vi "Save_Scan_macro.vi"(7 "Application":refnum<k7>, 8 "error in (no error)":errorcluster, 9 "InkScape":string, 10 "BMP INK Path":string, 11 "BMP Path":string) -> (0 "error out":errorcluster, 3 "BMP":picture)   [LabVIEW 2016]
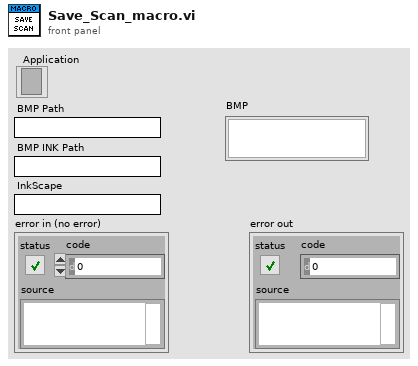
[diagram p1: front panel]
types:
  T1 = cluster{"CenterPosX":dbl, "CenterPosY":dbl, "ImageHeight":dbl, "ImageWidth":dbl}
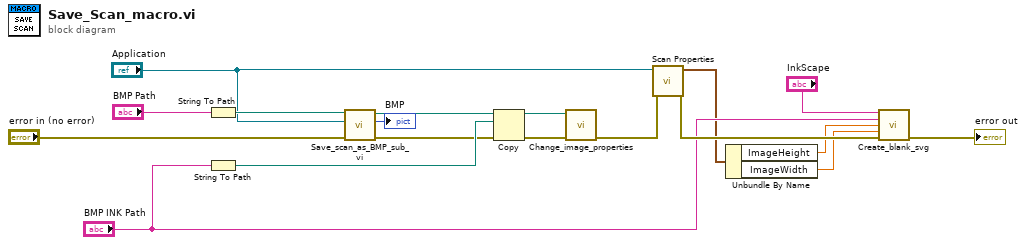
[diagram p0: block diagram]
diagram:
  n1 = String To Path(string="BMP Path") -> (path=w16:path)
  n2 = String To Path(string="BMP INK Path") -> (path=w14:path)
  n3 = call "Save_scan_as_BMP_sub_vi.vi"("error in (no error)"="error in (no error)", "Application"="Application", "BMP Path In"=w16) -> ("Error Out"=w13:errorcluster, "BMP"=→"BMP":picture, "BMP Path Out"=w18:path)  [unwired: 6 in]
  n4 = Copy(8:w13, 10:w14, 11:w18) -> (0:w12:errorcluster, 3:w15:path)  [unwired: 2 in, 1 out]
  n5 = call "Change_image_properties.vi"("error in (no error)"=w12, "Path In"=w15) -> ("error out"=w11:errorcluster)  [unwired: 8 in, 1 out]
  n6 = call "Scan Properties.vi"("error in (no error)"=w11, "Application"="Application") -> ("error out"=w10:errorcluster, "Scan Properties"=w7:T1)  [unwired: 8 in]
  n7 = Unbundle By Name(w7) -> ("ImageHeight"=w6:dbl, "ImageWidth"=w5:dbl)
  n8 = call "Create_blank_svg.vi"("SVG Path"="InkScape", "BMP for inkscape path"="BMP INK Path", "HEIGHT"=w6, "WIDTH"=w5, "error in"=w10) -> ("error out"=→"error out":errorcluster)  [unwired: 9 in, 1 out]
